vi "RS232C_Move_re.vi"(0 "Port Number":i8 min=0, 1 "Axis Count":u8=2, 2 "Axis Number":u8(ring)=1 items=["0", "1", "2", "3", "4"], 3 "Pulse Number":u32=100 min=1 max=500000, 4 "Direction":bool=TRUE, 5 "Delimiter":string="\\r\\n\r\n", 6 "Main/Sub":bool=TRUE) -> (7 "String Received":string, 8 "OK Done":bool)   [LabVIEW 2016]
panel:
  out "Command String":string
  out "Received String2":string
  # "Port Number 0=COM1"
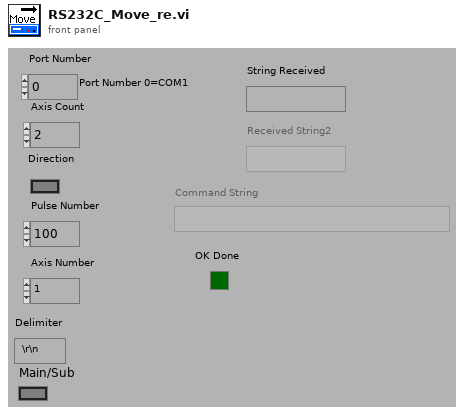
[diagram p1: front panel]
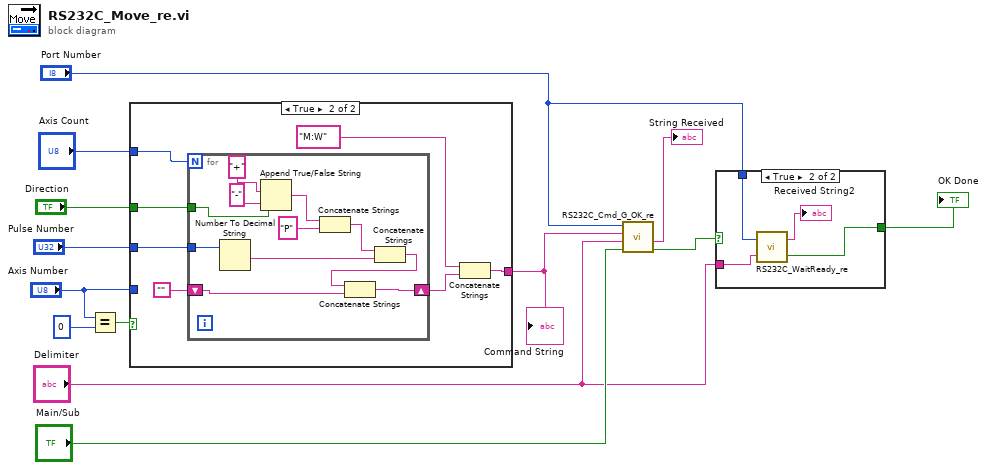
[diagram p0: block diagram]
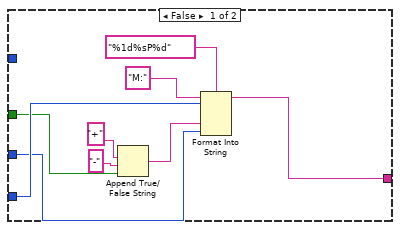
[diagram p2: hidden frame]
diagram:
  n1 = Equal?(x="Axis Number", y=0) -> (x = y?=w11:bool)
  n2 = case shown="True" w11 {
    tunnel: "Pulse Number" -> [w17 w28]
    tunnel: "Axis Number" -> [w18 _]
    tunnel: "Direction" -> [w16 w29]
    tunnel: [w14 w25] -> w3
    tunnel: "Axis Count" -> [_ w23]
    frame False {
      n3 = Append True/False String(1:w16, 2:"-", 3:"+") -> (0:w22:string)  [unwired: 1 out]
      n4 = Format Into String(format string="%1d%sP%d", initial string="M:", w18, w22, w17) -> (resulting string=w14:string)  [unwired: 1 in, 1 out]
    }
    frame True {
      n5 = for {
        N: w23 -> [_]
        tunnel: w29 -> [w38]
        tunnel: w28 -> [w35]
        shift-right: [w30] -> w26
        shift-left: "" -> [w31]
        n6 = Number To Decimal String(number=w35) -> (decimal integer string=w33:string)  [unwired: 1 in]
        n7 = Append True/False String(1:w38, 2:"-", 3:"+") -> (0:w37:string)  [unwired: 1 out]
        n8 = Concatenate Strings(w37, "P" ("文字列")) -> (w34:string)
        n9 = Concatenate Strings(w34, w33) -> (w32:string)
        n10 = Concatenate Strings(w32, w31) -> (w30:string)
      }
      n11 = Concatenate Strings("M:W", w26) -> (w25:string)
    }
  }
  "Command String" <- w3
  n12 = call "RS232C_Cmd_G_OK_re.vi"("Main/Sub"="Main/Sub", "Delimiter"="Delimiter", "Command String"=w3, "PortNumber"="Port Number") -> ("OK Done"=w5:bool, "Received String3"=→"String Received":string)  [unwired: 2 out]
  n13 = case shown="True" w5 {
    selector: w5 -> [w41 _]
    tunnel: "Port Number" -> [_ w44]
    tunnel: [w41 w45] -> w13
    tunnel: "Delimiter" -> [_ w42]
    frame False {
    }
    frame True {
      n14 = call "RS232C_WaitReady_re.vi"("Delimiter"=w42, "PortNumber"=w44) -> ("OK Done"=w45:bool, "String Received"=→"Received String2":string)
    }
  }
  "OK Done" <- w13
